vi "creat new file.vi"(3 "error in (no error)":errorcluster caption="错误输入（无错误）", 4 "file name":string, 5 "path":path) -> (0 "error out":errorcluster, 1 "file or folder exists?":bool caption="文件或文件夹存在？", 2 "created path":path)   [LabVIEW 2014]
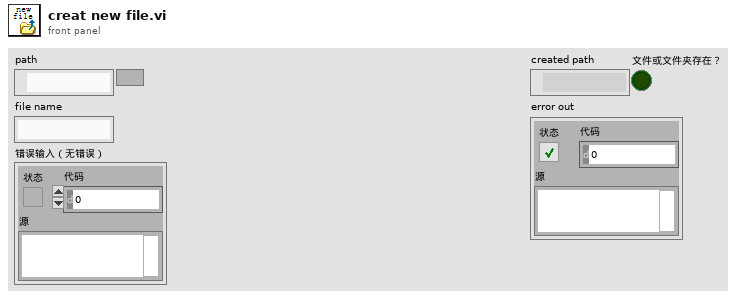
[diagram p1: front panel]
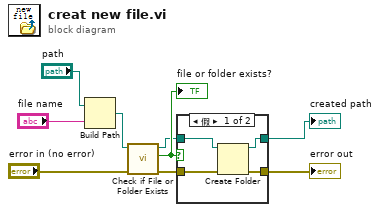
[diagram p0: block diagram]
diagram:
  n1 = Build Path(base path="path", name or relative path="file name") -> (appended path=w7:path)
  n2 = call <vilib>:"Check if File or Folder Exists.vi"("error in (no error)"="error in (no error)", "path"=w7) -> ("error out"=w2:errorcluster, "file or folder exists?"=w5:bool, "dup path"=w4:path)  [unwired: 7 in]
  "file or folder exists?" <- w5
  n3 = case shown="假" w5 {
    tunnel: [w10 w15] -> w3
    tunnel: w4 -> [w13 w15]
    tunnel: [w11 w14] -> w1
    tunnel: w2 -> [w12 w14]
    frame False {
      n4 = Create Folder(path (use dialog)=w13, error in=w12) -> (created path=w10:path, error out=w11:errorcluster)  [unwired: 1 in, 1 out]
    }
    frame True {
    }
  }
  "created path" <- w3
  "error out" <- w1
